vi "onListenForNewConnection.vi"(8 "error in (no error)":errorcluster, 9 "timeout (ms)":i32=1, 11 "Listener":refnum<class "Connection.NetworkStream.lvclass">) -> (0 "error out":errorcluster, 1 "New connection":bool, 2 "timed out":bool, 3 "New Connection":refnum<class "Connection.lvclass">)   [LabVIEW 2013]
uses:
  Connection.NetworkStream/Connection.NetworkStream.lvclass
  Connection/Connection.lvclass
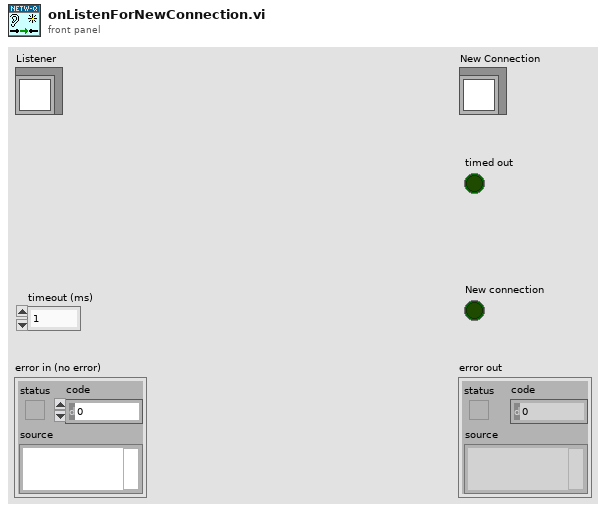
[diagram p1: front panel]
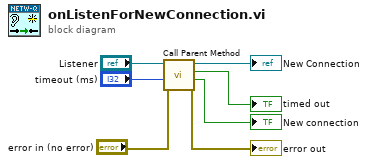
[diagram p0: block diagram]
diagram:
  n1 = call-parent "Call Parent Method"("error in (no error)"="error in (no error)", "timeout (ms)"="timeout (ms)", "Listener"="Listener") -> ("error out"=→"error out":errorcluster, "New connection"=→"New connection":bool, "timed out"=→"timed out":bool, "New Connection"=→"New Connection":refnum<class "Connection.lvclass">)  [unwired: 5 in]
